vi "ENVIA VALORES-SERVER.vi"() -> ()   [LabVIEW 2019]
uses:
  Strict_Type_Def_Valores_Instrumentos.ctl
  <vilib>/Utility/file.llb/Read Delimited Spreadsheet (string).vi
  Variaveis_Globais_CLP_Paralelo.vi
  Acionamento_Adquiri.vi
panel:
  in  "DP_Lam_max [mmCA]":bool
  in  "Q_Lam[m³/h]":dbl format="%#_4e"
  in  "Rho_Lam/Rho*":dbl
  in  "Mu*/Mu_Lam":dbl format="%#_4e"
  in  "Q*[m³/h]":dbl
  in  "M_Lam[Kg/h]":dbl
  in  "DP_Lam[mmCA]":dbl format="%#_4e"
  in  "SKM-PI-LAM":dbl format="%#_4e"
  in  "SMA-TI-LAM":dbl
  in  "SMA-PI-LAM":dbl
  in  "SKM-PI-BAR":dbl format="%#_4e"
  in  "SKM-TI-WF":dbl
  in  "SKM-TI-KF":dbl
  in  "SKM-TI-AR_COR":dbl
  in  "JK":dbl format="%#_4e"
  in  "JW":dbl format="%#_4e"
  in  "JL":dbl format="%#_4e"
  in  "JG":dbl
  in  "ADQ":bool
  out "size(s)":i32
  in  "SKM-FC-WF_MAX":dbl
  in  "SKM-FC-WF_MIN":dbl
  in  "SKM-PC-TQ_MAX":dbl
  in  "SKM-PC-TQ_MIN":dbl
  in  "SKM-FC-AR_MAX":dbl
  in  "SKM-FC-AR_MIN":dbl
  in  "SKM-FC-KF_MAX":dbl
  in  "SKM-FC-KF_MIN":dbl
  in  "SPK-WR-VEL_MAX":dbl
  in  "SPK-WR-VEL_MIN":dbl
  in  "SPW-WR-VEL_MIN":dbl
  in  "SPW-WR-VEL_MAX":dbl
  in  "SPK-INV-001_ON":bool
  in  "SPK-INV-001_OFF":bool
  in  "SPK-NC-CV-001":bool
  in  "SPK-NC-CV-002":bool
  in  "SPK-NC-CV-003":bool
  in  "SPK-NO-CV-005":bool
  in  "SPK-NC-CV-004":bool
  in  "SPK-NO-CV-006":bool
  in  "SPK-NO-CV-008":bool
  in  "SPK-NO-CV-007":bool
  in  "SPW-INV-001_OFF":bool
  in  "SPW-NC-CV-002":bool
  in  "SPW-INV-001_ON":bool
  in  "SPW-NC-CV-003":bool
  in  "SPW-NO-CV-006":bool
  in  "SPW-NC-CV-001":bool
  in  "SPW-NO-CV-005":bool
  in  "SPW-NO-CV-008":bool
  in  "SPW-NC-CV-004":bool
  in  "SPW-NO-CV-007":bool
  in  "SPW-WR-VEL":dbl
  in  "SPK-WR-VEL":dbl
  in  "SKM-NC-CV_COR":bool
  in  "SKM-NC-CV-JMP":bool
  in  "SKM-NC-CV-LAM":bool
  in  "SKM-FC-AR":dbl
  in  "SKM-FC-KF":dbl
  in  "SKM-FC-WF":dbl
  in  "SKM-PC-TQ":dbl
  in  "PC-TQ-ON":bool
  in  "SKM-AI-KF_COR":dbl
  in  "Diametro_tubulacao":dbl
  in  "SKM-FIC-KF_COR":dbl
  in  "SKM-FI-WF":dbl
  in  "SIA-NC-CV-001":bool
  in  "SIK-NC-CV-001":bool
  in  "SIK-NC-CV-002":bool
  in  "SIT-NC-CV-001":bool
  in  "SIT-NC-CV-002":bool
  in  "SIW-NC-CV-001":bool
  in  "SIW-NC-CV-002":bool
  in  "SKS-NC-CV-001":bool
  in  "SKS-NC-CV-002":bool
  in  "SKS-NC-CV-003":bool
  in  "SKS-NC-CV-004":bool
  in  "SKS-NC-CV-005":bool
  in  "SKS-NC-CV-006":bool
  in  "Valores_Instrumentos":T1 {"JG_AR" format="%#_6e"; "DeltaP_K" format="%#_6e"; "DeltaP_W" format="%#_6e"; "Diâmetro Tubulação [m]" format="%#_6e"; "PC-TQ-TD" format="%#_6e"; "PC-TQ-TI" format="%#_6e"; "PC-TQ-GP" format="%#_6e"; "PC-TQ-PV" format="%#_6e"; "PC-TQ-SP" format="%#_6e"; "PC-TQ-OV" format="%#_6e"; "SPW-WR-VEL" format="%#_6e"; "SPK-WR-VEL" format="%#_6e"; "SKM-PC-TQ" format="%#_6e"; "SKM-FC-KF" format="%#_6e"; "SKM-FC-WF" format="%#_6e"; "SKM-FC-AR" format="%#_6e"; "SKM-TI-KF_COR" format="%#_6e"; "SKS-LC-K" format="%#_6e"; "SPK-RD-CRT" format="%#_6e"; "SPW-RD-CRT" format="%#_6e"; "SKM-FIC-AR_COR" format="%#_6e"; "SKM-FIC-KF_COR" format="%#_6e"; "SKM-AI-AR_COR" format="%#_6e"; "SKM-AI-KF_COR" format="%#_6e"; "SKM-TI-AR_COR" format="%#_6e"; "SKM-TI-KF" format="%#_6e"; "SPW-RD-VEL" format="%#_6e"; "SPK-RD-VEL" format="%#_6e"; "SKS-LC-W" format="%#_6e"; "SIT-PI-002" format="%#_6e"; "SKM-FI-WF" format="%#_6e"; "SKM-TI-WF" format="%#_6e"; "SKM-PI-BAR" format="%#_6e"; "SKM-PI-LAM" format="%#_6e"; "SMA-PI-LAM" format="%#_6e"; "SMA-TI-LAM" format="%#_6e"; "SKM-PI-TQ" format="%#_6e"; "SKM-TI-TQ" format="%#_6e"}
  in  "stop":bool
  in  "VALORES VAZIOS":string[](array[string])
  out "RAN":dbl
  in  "FRA":string
  in  "FLO":dbl
  in  "NUM":i32
  in  "BOTAO":bool
  in  "NOMES":string[](array[string])
  out "Controles":cluster{refnum<vi>[]}
  out "VALORES":string[](array[string])
  # "SKID MEDI敲O - LEITURA"
  # "SKID MEDI敲O - ESCRITA"
  # "SKID BOMBA - ESCRITA"
  # "SKID BOMBA - LEITURA"
  # "SKID SEPARA敲O - LEITURA"
  # "SKID INJE敲O - LEITURA"
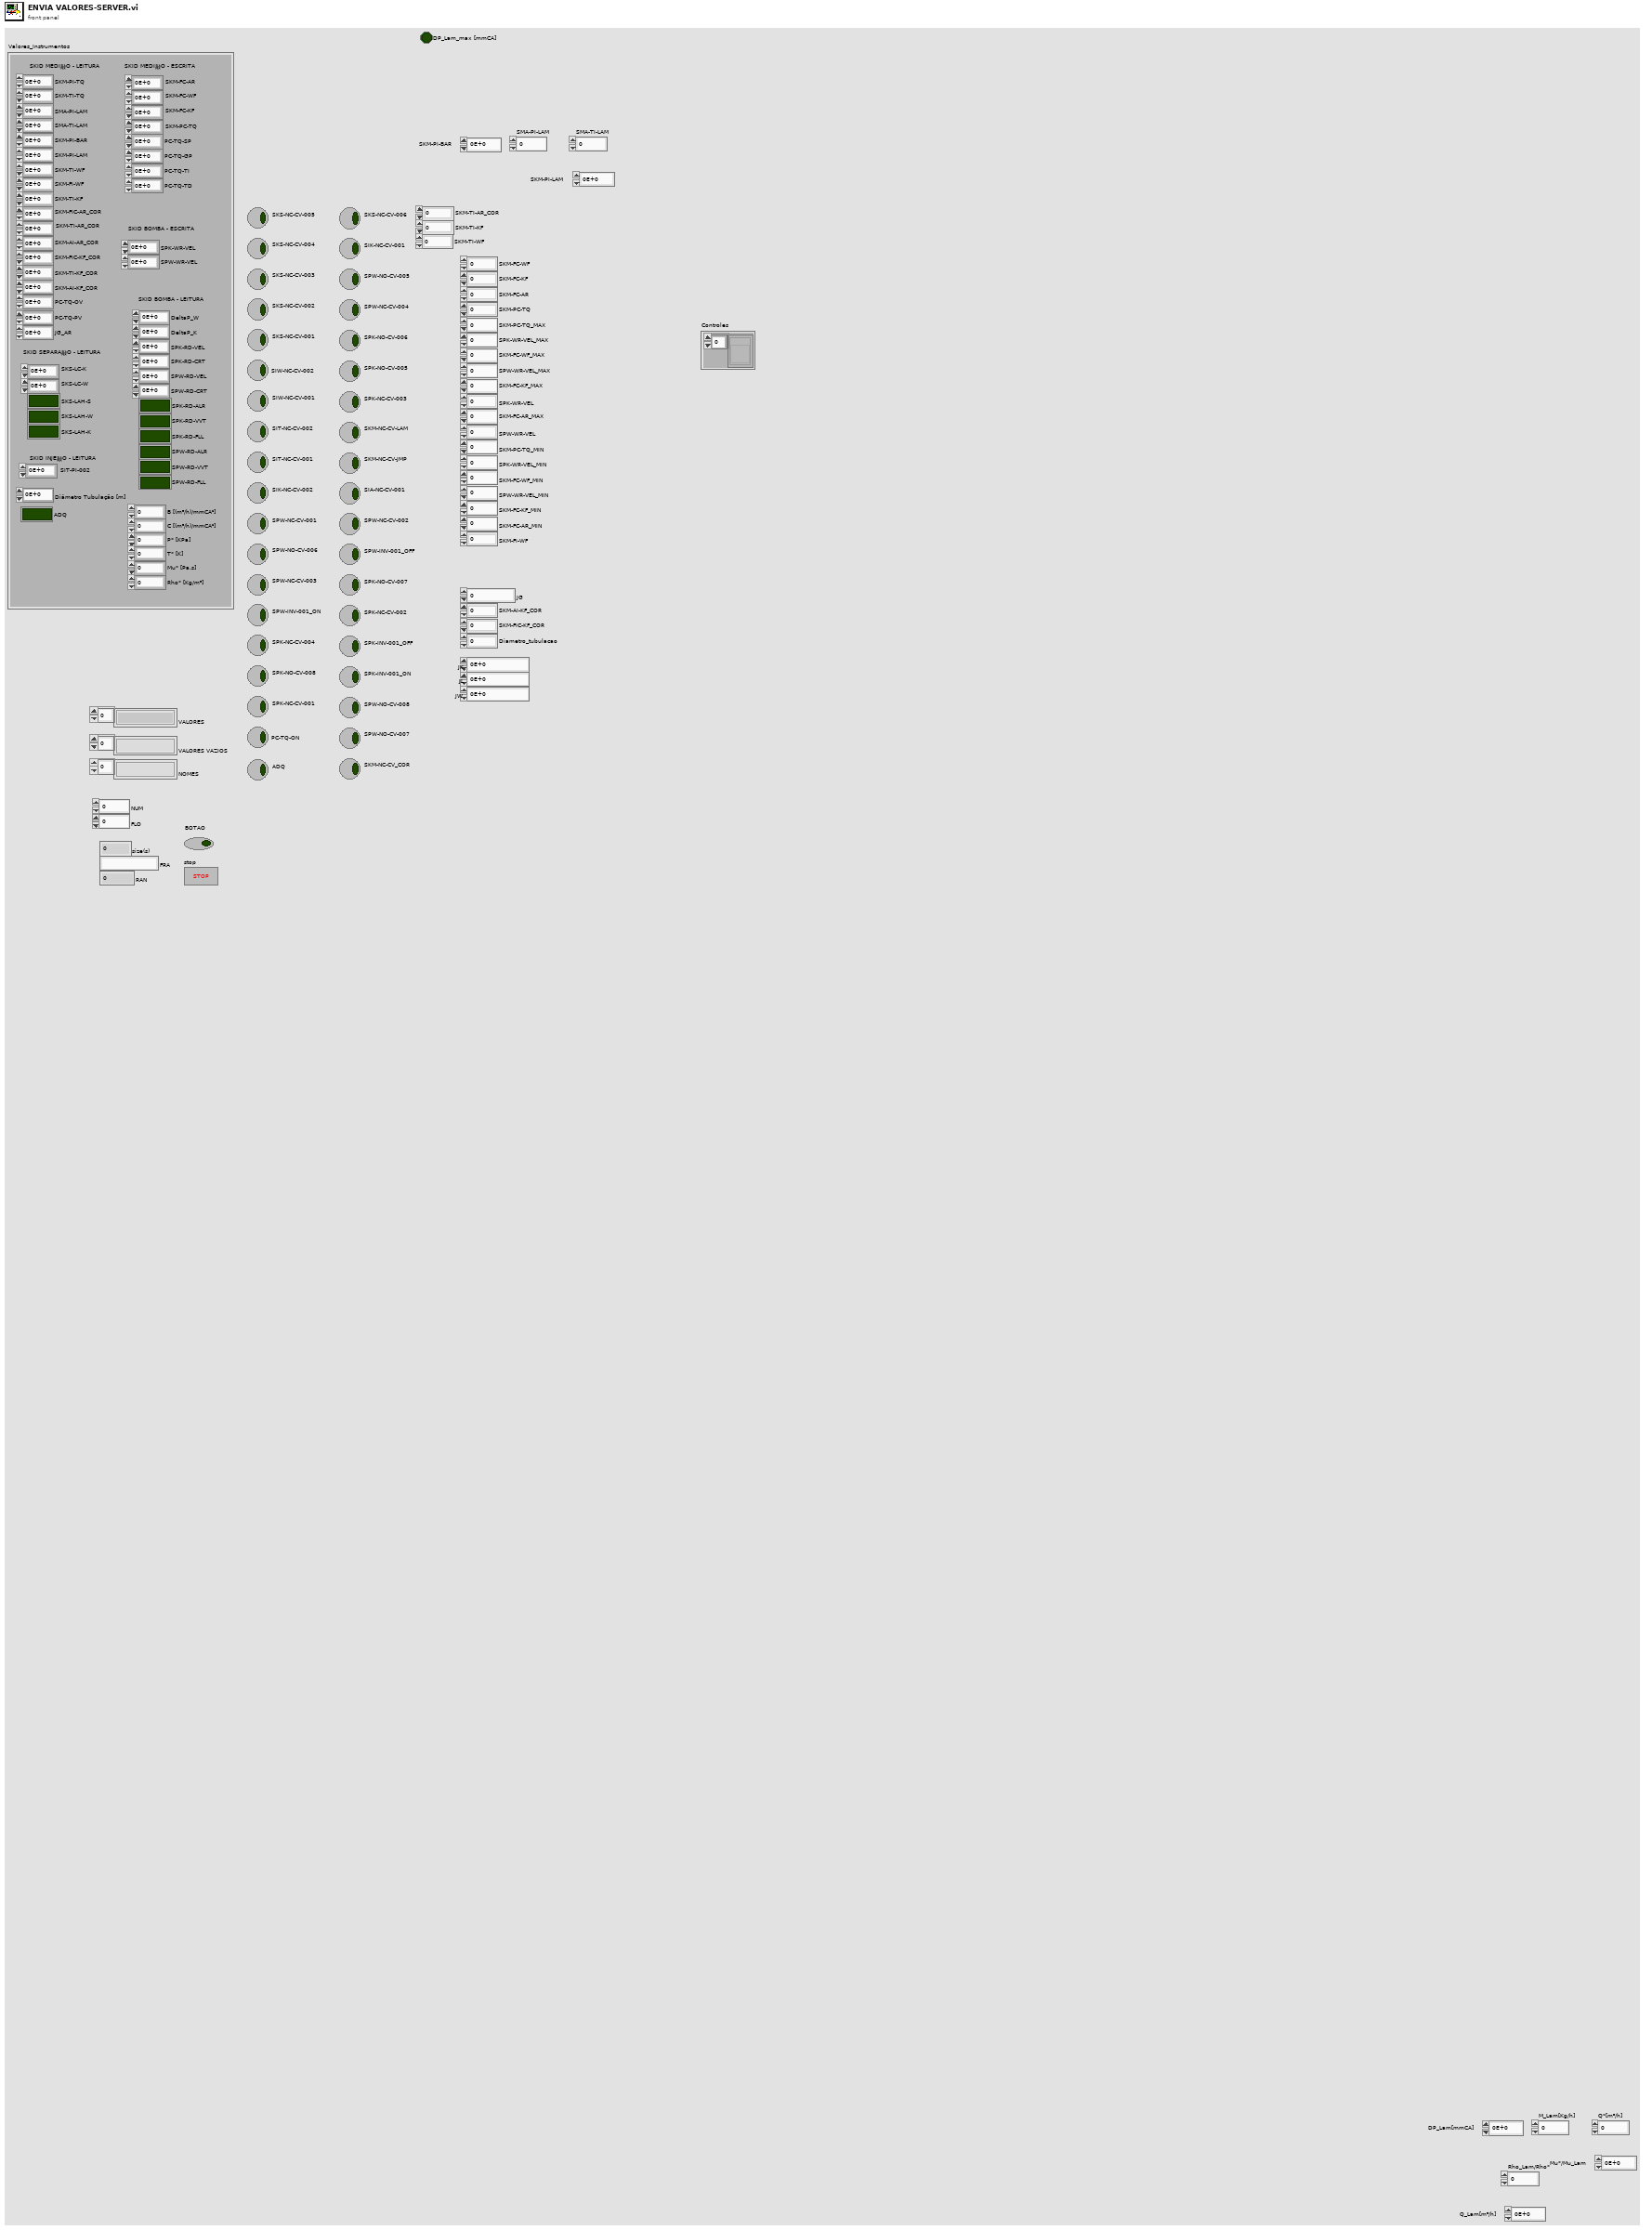
[diagram p1: front panel]
types:
  T1 = typedef "Strict_Type_Def_Valores_Instrumentos.ctl" = cluster{"SKM-TI-TQ":dbl, "SKM-PI-TQ":dbl, "SMA-TI-LAM":dbl, "SMA-PI-LAM":dbl, "SKM-PI-LAM":dbl, "SKM-PI-BAR":dbl, "SKM-TI-WF":dbl, "SKM-FI-WF":dbl, "SIT-PI-002":dbl, "SKS-LC-W":dbl, "SPK-RD-VEL":dbl, "SPW-RD-VEL":dbl, "SKM-TI-KF":dbl, "SKM-TI-AR_COR":dbl, "SKM-AI-KF_COR":dbl, "SKM-AI-AR_COR":dbl, "SKM-FIC-KF_COR":dbl, "SKM-FIC-AR_COR":dbl, "SPW-RD-CRT":dbl, "SPK-RD-CRT":dbl, "SKS-LC-K":dbl, "SKM-TI-KF_COR":dbl, "SKM-FC-AR":dbl, "SKM-FC-WF":dbl, "SKM-FC-KF":dbl, "SKM-PC-TQ":dbl, "SPK-WR-VEL":dbl, "SPW-WR-VEL":dbl, "SPK-RD-ALR":bool, "SPK-RD-VVT":bool, "SPK-RD-FLL":bool, "SPW-RD-ALR":bool, "SPW-RD-VVT":bool, "SPW-RD-FLL":bool, "PC-TQ-OV":dbl, "PC-TQ-SP":dbl, "PC-TQ-PV":dbl, "PC-TQ-GP":dbl, "PC-TQ-TI":dbl, "PC-TQ-TD":dbl, "SKS-LAH-S":bool, "SKS-LAH-W":bool, "SKS-LAH-K":bool, "Diâmetro Tubulação [m]":dbl, "DeltaP_W":dbl, "DeltaP_K":dbl, "ADQ":bool, "JG_AR":dbl, "B [(m³/h)/mmCA²]":dbl, "C [(m³/h)/mmCA²]":dbl, "P* [KPa]":dbl, "T* [K]":dbl, "Mu* [Pa.s] ":dbl, "Rho* [Kg/m³]":dbl}
  T2 = cluster{"Application Name":string, "Description":string, "SPK-NC-CV-001":bool, "SPK-NC-CV-002":bool, "SPK-NC-CV-003":bool, "SPK-NC-CV-004":bool, "SPK-NO-CV-005":bool, "SPK-NO-CV-006":bool, "SPK-NO-CV-007":bool, "SPK-NO-CV-008":bool, "SPK-INV-001":bool, "SPW-NC-CV-001":bool, "SPW-NC-CV-002":bool, "SPW-NC-CV-003":bool, "SPW-NC-CV-004":bool, "SPW-NO-CV-005":bool, "SPW-NO-CV-006":bool, "SPW-NO-CV-007":bool, "SPW-NO-CV-008":bool, "SPW-INV-001":bool, "SKM-NC-CV-LAM":bool, "SKM-NC-CV-COR":bool, "SKM-FV-AR":bool, "SKM-PV-TQ":bool, "SKM-NC-CV-JMP":bool, "SKM-FV-WF":bool, "SKM-FV-KF":bool, "SIW-NC-CV-001":bool, "SIA-NC-CV-001":bool, "SIK-NC-CV-001":bool, "SIT-NC-CV-002":bool, "SIT-NC-CV-001":bool, "SIK-NC-CV-002":bool, "SIW-NC-CV-002":bool, "SKS-NC-CV-001":bool, "SKS-NC-CV-002":bool, "SKS-NC-CV-003":bool, "Boolean":bool, "Boolean 2":bool, "SKS-NC-CV-006":bool}
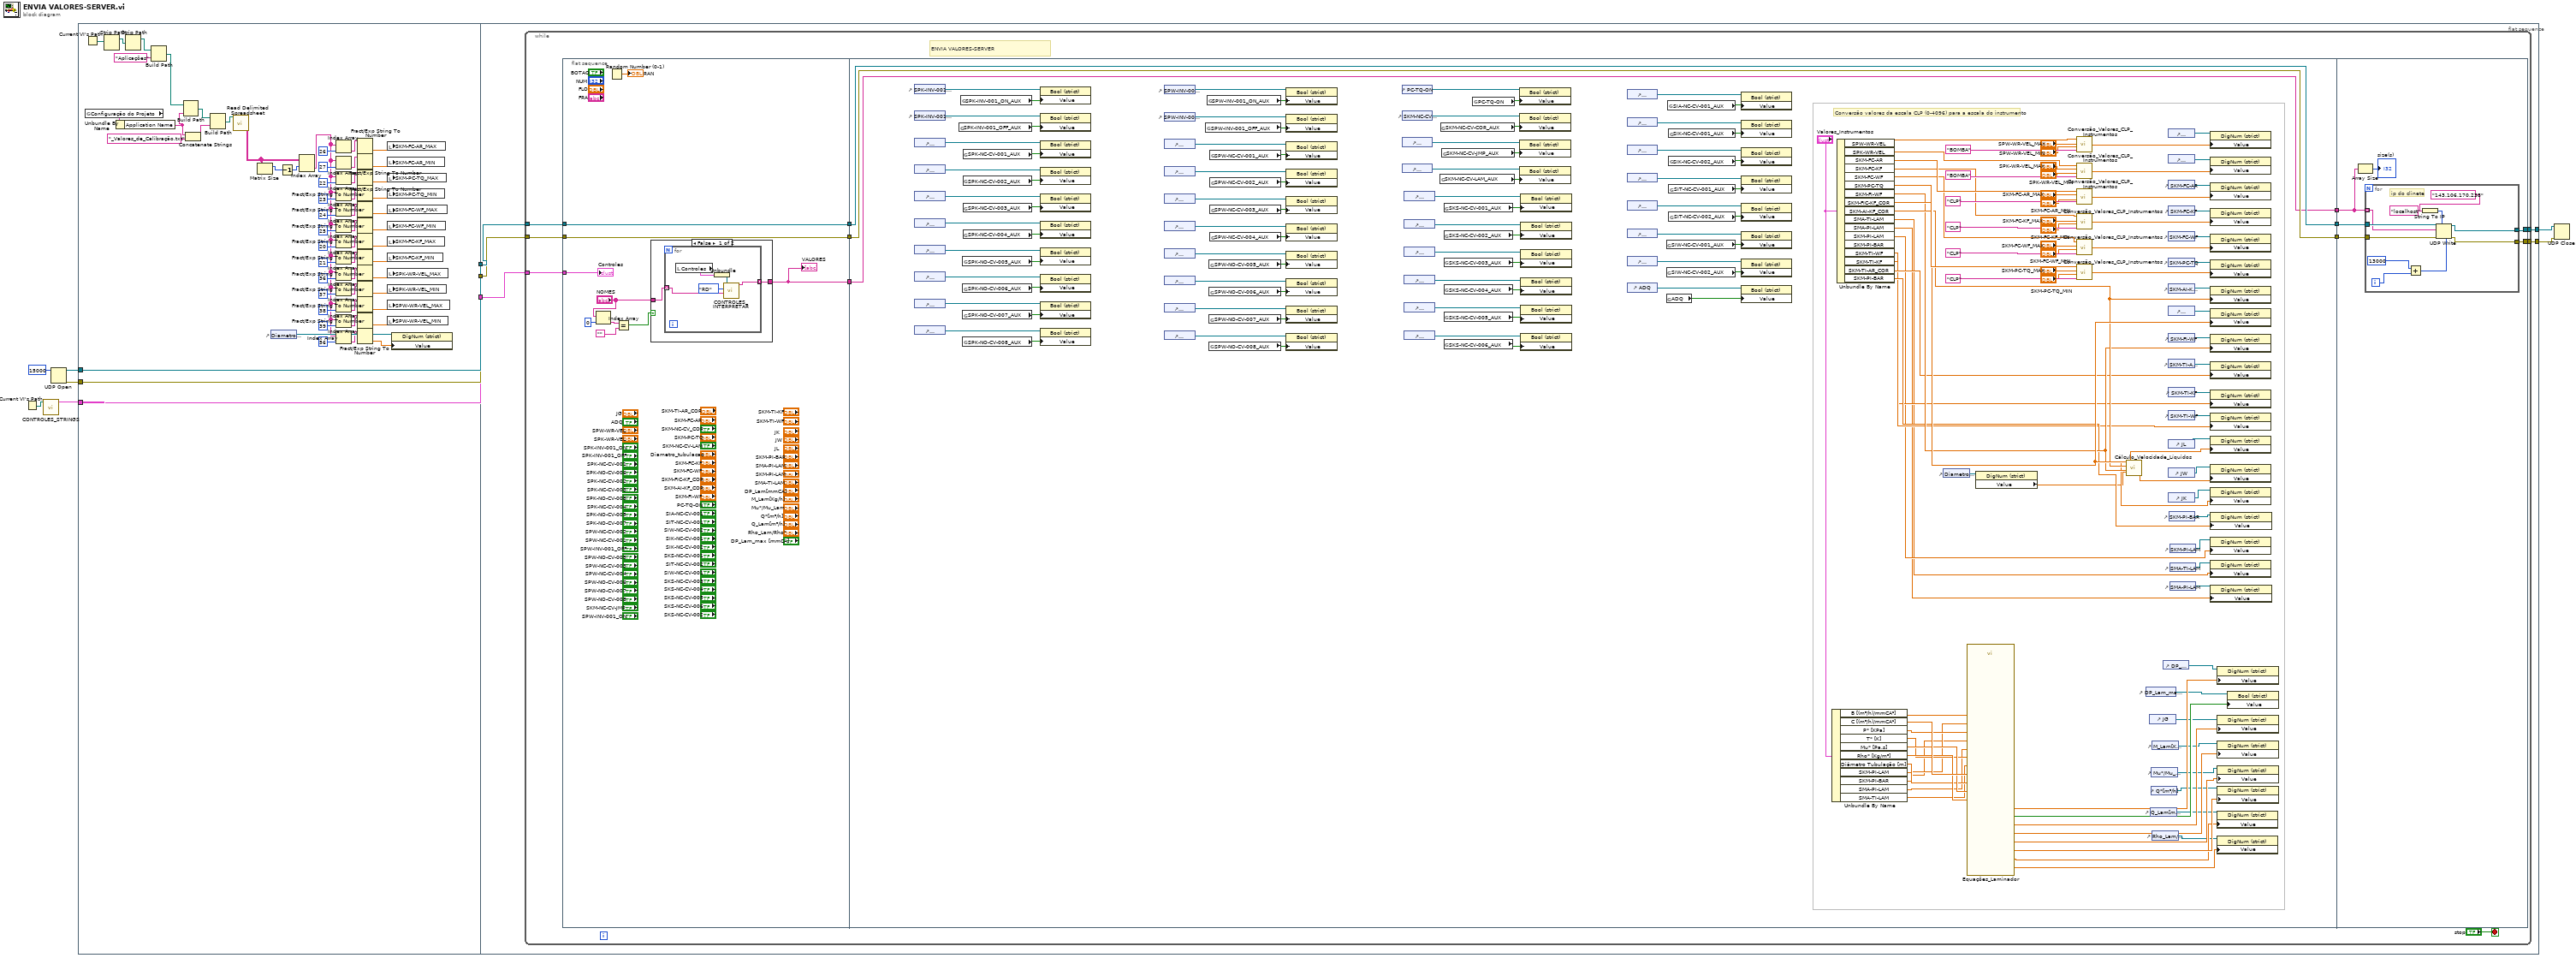
[diagram p0: block diagram]
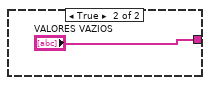
[diagram p2: hidden frame]
diagram:
  n1 = Current VI's Path() -> (path=w7:path)
  n2 = call "CONTROLES_STRINGS.vi"("vi path"=w7) -> ("output cluster"=w6:cluster{refnum<vi>[]})  [unwired: 9 in, 1 out]
  n3 = UDP Open(11:u16 15000 ("port")) -> (port=w9:refnum<k16>, 0:w8:errorcluster)  [unwired: 4 in, 1 out]
  n4 = flat-sequence {
    tunnel: w6 -> [w66]
    tunnel: w8 -> [w67]
    tunnel: w9 -> [w68]
    tunnel: [w68] -> w5
    tunnel: [w67] -> w4
    tunnel: [w66] -> w3
    tunnel: w5 -> [w70]
    tunnel: w4 -> [w69]
    tunnel: w3 -> [w73]
    tunnel: [w72] -> w2
    tunnel: [w71] -> w1
    frame #0 {
      n5 = Current VI's Path() -> (path=w65:path)
      n6 = global read "Variaveis_Globais_para_Configurar_Aplicação_Paralelo.vi" "Configuração do Projeto"() -> (w60:T2)
      n7 = Strip Path(path=w65) -> (stripped path=w64:path)  [unwired: 1 out]
      n8 = Unbundle By Name(w60) -> ("Application Name"=w57:string)
      n9 = Strip Path(path=w64) -> (stripped path=w63:path)  [unwired: 1 out]
      n10 = Build Path(base path=w63, name or relative path="Aplicações") -> (appended path=w61:path)
      n11 = Build Path(base path=w61, name or relative path=w57) -> (appended path=w59:path)
      n12 = Concatenate Strings(w57, "_Valores_de_Calibração.txt" ("string")) -> (w58:string)
      n13 = Build Path(base path=w59, name or relative path=w58) -> (appended path=w55:path)
      n14 = call-poly <vilib>:"Read Delimited Spreadsheet.vi"("file path (dialog if empty)"=w55) -> ("all rows"=w54:string[][])  [unwired: 9 in, 5 out]
      n15 = Matrix Size(0:w54) -> (1:w17:i32)  [unwired: 1 out]
      n16 = control-ref of="Diametro_tubulacao"() -> (w15:refnum<vi>)
      n17 = Decrement(x=w17) -> (x-1=w16:i32)
      n18 = Index Array(array=w54, index (row)=w16) -> (element=w11:string[])  [unwired: 1 in]
      n19 = Index Array(array=w11, index=26) -> (element=w46:string)
      n20 = Index Array(array=w11, index=27) -> (element=w47:string)
      n21 = Index Array(array=w11, index=22) -> (element=w48:string)
      n22 = Index Array(array=w11, index=23) -> (element=w49:string)
      n23 = Index Array(array=w11, index=24) -> (element=w44:string)
      n24 = Index Array(array=w11, index=25) -> (element=w43:string)
      n25 = Index Array(array=w11, index=20) -> (element=w42:string)
      n26 = Index Array(array=w11, index=21) -> (element=w41:string)
      n27 = Index Array(array=w11, index=36) -> (element=w40:string)
      n28 = Index Array(array=w11, index=37) -> (element=w39:string)
      n29 = Index Array(array=w11, index=38) -> (element=w38:string)
      n30 = Index Array(array=w11, index=39) -> (element=w37:string)
      n31 = Index Array(array=w11, index=56) -> (element=w13:string)
      n32 = Fract/Exp String To Number(string=w46) -> (number=w20:dbl)  [unwired: 3 in, 1 out]
      n33 = Fract/Exp String To Number(string=w47) -> (number=w19:dbl)  [unwired: 3 in, 1 out]
      n34 = Fract/Exp String To Number(string=w48) -> (number=w30:dbl)  [unwired: 3 in, 1 out]
      n35 = Fract/Exp String To Number(string=w49) -> (number=w29:dbl)  [unwired: 3 in, 1 out]
      n36 = Fract/Exp String To Number(string=w44) -> (number=w28:dbl)  [unwired: 3 in, 1 out]
      n37 = Fract/Exp String To Number(string=w43) -> (number=w27:dbl)  [unwired: 3 in, 1 out]
      n38 = Fract/Exp String To Number(string=w42) -> (number=w26:dbl)  [unwired: 3 in, 1 out]
      n39 = Fract/Exp String To Number(string=w41) -> (number=w25:dbl)  [unwired: 3 in, 1 out]
      n40 = Fract/Exp String To Number(string=w40) -> (number=w24:dbl)  [unwired: 3 in, 1 out]
      n41 = Fract/Exp String To Number(string=w39) -> (number=w23:dbl)  [unwired: 3 in, 1 out]
      n42 = Fract/Exp String To Number(string=w38) -> (number=w22:dbl)  [unwired: 3 in, 1 out]
      n43 = Fract/Exp String To Number(string=w37) -> (number=w21:dbl)  [unwired: 3 in, 1 out]
      n44 = Fract/Exp String To Number(string=w13) -> (number=w12:dbl)  [unwired: 3 in, 1 out]
      n45 = local write "SKM-FC-AR_MAX"(w20) -> ()
      n46 = local write "SKM-FC-AR_MIN"(w19) -> ()
      n47 = local write "SKM-PC-TQ_MAX"(w30) -> ()
      n48 = local write "SKM-PC-TQ_MIN"(w29) -> ()
      n49 = local write "SKM-FC-WF_MAX"(w28) -> ()
      n50 = local write "SKM-FC-WF_MIN"(w27) -> ()
      n51 = local write "SKM-FC-KF_MAX"(w26) -> ()
      n52 = local write "SKM-FC-KF_MIN"(w25) -> ()
      n53 = local write "SPK-WR-VEL_MAX"(w24) -> ()
      n54 = local write "SPK-WR-VEL_MIN"(w23) -> ()
      n55 = local write "SPW-WR-VEL_MAX"(w22) -> ()
      n56 = local write "SPW-WR-VEL_MIN"(w21) -> ()
      n57 = property class="DigNum (strict)"(reference=w15, "Value"=w12) -> ()  [unwired: 1 in, 2 out]
    }
    frame #1 {
      n58 = while {
        tunnel: w73 -> [w85]
        tunnel: [w77] -> w72
        tunnel: [w76] -> w71
        tunnel: w70 -> [w75]
        tunnel: w69 -> [w74]
        stop <- "stop" stop-if-true
        # "ENVIA VALORES-SERVER"
        n59 = flat-sequence {
          tunnel: [w95] -> w83
          tunnel: [w94] -> w81
          tunnel: [w93] -> w79
          tunnel: w75 -> [w95]
          tunnel: w74 -> [w94]
          tunnel: w85 -> [w91]
          tunnel: w83 -> [w274]
          tunnel: [w274] -> w82
          tunnel: w81 -> [w273]
          tunnel: [w273] -> w80
          tunnel: w79 -> [w272]
          tunnel: [w272] -> w78
          tunnel: [w278] -> w77
          tunnel: [w277] -> w76
          tunnel: w82 -> [w280]
          tunnel: w80 -> [w279]
          tunnel: w78 -> [w276]
          frame #0 {
            n60 = Index Array(array="NOMES", index=0) -> (element=w88:string)
            n61 = Random Number (0-1)() -> (number: 0 to 1=→"RAN":dbl)
            n62 = Equal?(x=w88, y="") -> (x = y?=w86:bool)
            n63 = case shown="False" w86 {
              tunnel: [w97 "VALORES VAZIOS"] -> w93
              tunnel: "NOMES" -> [w96 _]
              frame False {
                n64 = for {
                  tunnel: w96 -> [w100] mode=indexing
                  tunnel: [w98] -> w97 mode=indexing
                  n65 = local read "Controles"() -> (w102:cluster{refnum<vi>[]})
                  n66 = Unbundle(w102) -> (w101:refnum<vi>[])
                  n67 = call "CONTROLES_INTERPRETAR.vi"("name"=w100, "RD/WR"=enum16{"WR", "RD"}."RD", "Controls[]"=w101) -> ("Data"=w98:string)  [unwired: 6 in, 2 out]
                }
              }
              frame True {
              }
            }
            "VALORES" <- w93
            "Controles" <- w91
          }
          frame #1 {
            # "Conversão valores da escala CLP (0-4096) para a escala do instrumento"
            n68 = control-ref of="SPK-INV-001_ON"() -> (w253:refnum<vi>)
            n69 = control-ref of="SPK-INV-001_OFF"() -> (w254:refnum<vi>)
            n70 = control-ref of="SPK-NC-CV-001"() -> (w255:refnum<vi>)
            n71 = control-ref of="SPK-NC-CV-002"() -> (w256:refnum<vi>)
            n72 = control-ref of="SPK-NC-CV-003"() -> (w257:refnum<vi>)
            n73 = control-ref of="SPK-NC-CV-004"() -> (w259:refnum<vi>)
            n74 = control-ref of="SPK-NO-CV-005"() -> (w258:refnum<vi>)
            n75 = control-ref of="SPK-NO-CV-006"() -> (w260:refnum<vi>)
            n76 = control-ref of="SPK-NO-CV-007"() -> (w262:refnum<vi>)
            n77 = control-ref of="SPK-NO-CV-008"() -> (w261:refnum<vi>)
            n78 = global read "Variaveis_Globais_CLP_Paralelo.vi" "SPK-INV-001_OFF_AUX"() -> (w270:bool)
            n79 = global read "Variaveis_Globais_CLP_Paralelo.vi" "SPK-INV-001_ON_AUX"() -> (w271:bool)
            n80 = global read "Variaveis_Globais_CLP_Paralelo.vi" "SPK-NO-CV-005_AUX"() -> (w265:bool)
            n81 = global read "Variaveis_Globais_CLP_Paralelo.vi" "SPK-NO-CV-006_AUX"() -> (w264:bool)
            n82 = global read "Variaveis_Globais_CLP_Paralelo.vi" "SPK-NO-CV-007_AUX"() -> (w263:bool)
            n83 = global read "Variaveis_Globais_CLP_Paralelo.vi" "SPK-NO-CV-008_AUX"() -> (w160:bool)
            n84 = global read "Variaveis_Globais_CLP_Paralelo.vi" "SPK-NC-CV-001_AUX"() -> (w269:bool)
            n85 = global read "Variaveis_Globais_CLP_Paralelo.vi" "SPK-NC-CV-002_AUX"() -> (w268:bool)
            n86 = global read "Variaveis_Globais_CLP_Paralelo.vi" "SPK-NC-CV-003_AUX"() -> (w267:bool)
            n87 = global read "Variaveis_Globais_CLP_Paralelo.vi" "SPK-NC-CV-004_AUX"() -> (w266:bool)
            n88 = property class="Bool (strict)"(reference=w253, "Value"=w271) -> ()  [unwired: 1 in, 2 out]
            n89 = property class="Bool (strict)"(reference=w254, "Value"=w270) -> ()  [unwired: 1 in, 2 out]
            n90 = property class="Bool (strict)"(reference=w255, "Value"=w269) -> ()  [unwired: 1 in, 2 out]
            n91 = property class="Bool (strict)"(reference=w256, "Value"=w268) -> ()  [unwired: 1 in, 2 out]
            n92 = property class="Bool (strict)"(reference=w257, "Value"=w267) -> ()  [unwired: 1 in, 2 out]
            n93 = property class="Bool (strict)"(reference=w259, "Value"=w266) -> ()  [unwired: 1 in, 2 out]
            n94 = property class="Bool (strict)"(reference=w258, "Value"=w265) -> ()  [unwired: 1 in, 2 out]
            n95 = property class="Bool (strict)"(reference=w260, "Value"=w264) -> ()  [unwired: 1 in, 2 out]
            n96 = property class="Bool (strict)"(reference=w262, "Value"=w263) -> ()  [unwired: 1 in, 2 out]
            n97 = property class="Bool (strict)"(reference=w261, "Value"=w160) -> ()  [unwired: 1 in, 2 out]
            n98 = control-ref of="SPW-INV-001_ON"() -> (w235:refnum<vi>)
            n99 = control-ref of="SPW-INV-001_OFF"() -> (w233:refnum<vi>)
            n100 = control-ref of="SPW-NC-CV-001"() -> (w238:refnum<vi>)
            n101 = control-ref of="SPW-NC-CV-002"() -> (w234:refnum<vi>)
            n102 = control-ref of="SPW-NC-CV-003"() -> (w236:refnum<vi>)
            n103 = control-ref of="SPW-NC-CV-004"() -> (w241:refnum<vi>)
            n104 = control-ref of="SPW-NO-CV-005"() -> (w239:refnum<vi>)
            n105 = control-ref of="SPW-NO-CV-006"() -> (w237:refnum<vi>)
            n106 = control-ref of="SPW-NO-CV-007"() -> (w242:refnum<vi>)
            n107 = control-ref of="SPW-NO-CV-008"() -> (w240:refnum<vi>)
            n108 = global read "Variaveis_Globais_CLP_Paralelo.vi" "SPW-INV-001_OFF_AUX"() -> (w243:bool)
            n109 = global read "Variaveis_Globais_CLP_Paralelo.vi" "SPW-INV-001_ON_AUX"() -> (w245:bool)
            n110 = global read "Variaveis_Globais_CLP_Paralelo.vi" "SPW-NO-CV-005_AUX"() -> (w249:bool)
            n111 = global read "Variaveis_Globais_CLP_Paralelo.vi" "SPW-NO-CV-006_AUX"() -> (w247:bool)
            n112 = global read "Variaveis_Globais_CLP_Paralelo.vi" "SPW-NO-CV-007_AUX"() -> (w252:bool)
            n113 = global read "Variaveis_Globais_CLP_Paralelo.vi" "SPW-NO-CV-008_AUX"() -> (w250:bool)
            n114 = global read "Variaveis_Globais_CLP_Paralelo.vi" "SPW-NC-CV-001_AUX"() -> (w248:bool)
            n115 = global read "Variaveis_Globais_CLP_Paralelo.vi" "SPW-NC-CV-002_AUX"() -> (w244:bool)
            n116 = global read "Variaveis_Globais_CLP_Paralelo.vi" "SPW-NC-CV-003_AUX"() -> (w246:bool)
            n117 = global read "Variaveis_Globais_CLP_Paralelo.vi" "SPW-NC-CV-004_AUX"() -> (w251:bool)
            n118 = property class="Bool (strict)"(reference=w235, "Value"=w245) -> ()  [unwired: 1 in, 2 out]
            n119 = property class="Bool (strict)"(reference=w233, "Value"=w243) -> ()  [unwired: 1 in, 2 out]
            n120 = property class="Bool (strict)"(reference=w238, "Value"=w248) -> ()  [unwired: 1 in, 2 out]
            n121 = property class="Bool (strict)"(reference=w234, "Value"=w244) -> ()  [unwired: 1 in, 2 out]
            n122 = property class="Bool (strict)"(reference=w236, "Value"=w246) -> ()  [unwired: 1 in, 2 out]
            n123 = property class="Bool (strict)"(reference=w241, "Value"=w251) -> ()  [unwired: 1 in, 2 out]
            n124 = property class="Bool (strict)"(reference=w239, "Value"=w249) -> ()  [unwired: 1 in, 2 out]
            n125 = property class="Bool (strict)"(reference=w237, "Value"=w247) -> ()  [unwired: 1 in, 2 out]
            n126 = property class="Bool (strict)"(reference=w242, "Value"=w252) -> ()  [unwired: 1 in, 2 out]
            n127 = property class="Bool (strict)"(reference=w240, "Value"=w250) -> ()  [unwired: 1 in, 2 out]
            n128 = control-ref of="PC-TQ-ON"() -> (w228:refnum<vi>)
            n129 = control-ref of="SKM-NC-CV_COR"() -> (w225:refnum<vi>)
            n130 = control-ref of="SKM-NC-CV-JMP"() -> (w226:refnum<vi>)
            n131 = control-ref of="SKM-NC-CV-LAM"() -> (w227:refnum<vi>)
            n132 = control-ref of="SKS-NC-CV-001"() -> (w214:refnum<vi>)
            n133 = control-ref of="SKS-NC-CV-002"() -> (w215:refnum<vi>)
            n134 = control-ref of="SKS-NC-CV-003"() -> (w216:refnum<vi>)
            n135 = control-ref of="SKS-NC-CV-004"() -> (w217:refnum<vi>)
            n136 = control-ref of="SKS-NC-CV-005"() -> (w218:refnum<vi>)
            n137 = control-ref of="SKS-NC-CV-006"() -> (w213:refnum<vi>)
            n138 = global read "Variaveis_Globais_CLP_Paralelo.vi" "SKM-NC-CV-LAM_AUX"() -> (w229:bool)
            n139 = global read "Variaveis_Globais_CLP_Paralelo.vi" "SKM-NC-CV-COR_AUX"() -> (w231:bool)
            n140 = global read "Variaveis_Globais_CLP_Paralelo.vi" "SKM-NC-CV-JMP_AUX"() -> (w230:bool)
            n141 = global read "Variaveis_Globais_CLP_Paralelo.vi" "SKS-NC-CV-001_AUX"() -> (w219:bool)
            n142 = global read "Variaveis_Globais_CLP_Paralelo.vi" "SKS-NC-CV-002_AUX"() -> (w224:bool)
            n143 = global read "Variaveis_Globais_CLP_Paralelo.vi" "SKS-NC-CV-003_AUX"() -> (w223:bool)
            n144 = global read "Variaveis_Globais_CLP_Paralelo.vi" "SKS-NC-CV-004_AUX"() -> (w222:bool)
            n145 = global read "Variaveis_Globais_CLP_Paralelo.vi" "SKS-NC-CV-005_AUX"() -> (w221:bool)
            n146 = global read "Variaveis_Globais_CLP_Paralelo.vi" "SKS-NC-CV-006_AUX"() -> (w220:bool)
            n147 = global read "Variaveis_Globais_CLP_Paralelo.vi" "PC-TQ-ON"() -> (w232:bool)
            n148 = property class="Bool (strict)"(reference=w228, "Value"=w232) -> ()  [unwired: 1 in, 2 out]
            n149 = property class="Bool (strict)"(reference=w225, "Value"=w231) -> ()  [unwired: 1 in, 2 out]
            n150 = property class="Bool (strict)"(reference=w226, "Value"=w230) -> ()  [unwired: 1 in, 2 out]
            n151 = property class="Bool (strict)"(reference=w227, "Value"=w229) -> ()  [unwired: 1 in, 2 out]
            n152 = property class="Bool (strict)"(reference=w214, "Value"=w219) -> ()  [unwired: 1 in, 2 out]
            n153 = property class="Bool (strict)"(reference=w215, "Value"=w224) -> ()  [unwired: 1 in, 2 out]
            n154 = property class="Bool (strict)"(reference=w216, "Value"=w223) -> ()  [unwired: 1 in, 2 out]
            n155 = property class="Bool (strict)"(reference=w217, "Value"=w222) -> ()  [unwired: 1 in, 2 out]
            n156 = property class="Bool (strict)"(reference=w218, "Value"=w221) -> ()  [unwired: 1 in, 2 out]
            n157 = property class="Bool (strict)"(reference=w213, "Value"=w220) -> ()  [unwired: 1 in, 2 out]
            n158 = control-ref of="SIA-NC-CV-001"() -> (w199:refnum<vi>)
            n159 = control-ref of="SIK-NC-CV-001"() -> (w200:refnum<vi>)
            n160 = control-ref of="SIK-NC-CV-002"() -> (w201:refnum<vi>)
            n161 = control-ref of="SIT-NC-CV-001"() -> (w202:refnum<vi>)
            n162 = control-ref of="SIT-NC-CV-002"() -> (w203:refnum<vi>)
            n163 = control-ref of="SIW-NC-CV-001"() -> (w204:refnum<vi>)
            n164 = control-ref of="SIW-NC-CV-002"() -> (w205:refnum<vi>)
            n165 = control-ref of="ADQ"() -> (w159:refnum<vi>)
            n166 = global read "Variaveis_Globais_CLP_Paralelo.vi" "SIW-NC-CV-001_AUX"() -> (w207:bool)
            n167 = global read "Variaveis_Globais_CLP_Paralelo.vi" "SIW-NC-CV-002_AUX"() -> (w206:bool)
            n168 = global read "Acionamento_Adquiri.vi" "ADQ"() -> (w158:bool)
            n169 = global read "Variaveis_Globais_CLP_Paralelo.vi" "SIA-NC-CV-001_AUX"() -> (w212:bool)
            n170 = global read "Variaveis_Globais_CLP_Paralelo.vi" "SIK-NC-CV-001_AUX"() -> (w211:bool)
            n171 = global read "Variaveis_Globais_CLP_Paralelo.vi" "SIK-NC-CV-002_AUX"() -> (w210:bool)
            n172 = global read "Variaveis_Globais_CLP_Paralelo.vi" "SIT-NC-CV-001_AUX"() -> (w209:bool)
            n173 = global read "Variaveis_Globais_CLP_Paralelo.vi" "SIT-NC-CV-002_AUX"() -> (w208:bool)
            n174 = property class="Bool (strict)"(reference=w199, "Value"=w212) -> ()  [unwired: 1 in, 2 out]
            n175 = property class="Bool (strict)"(reference=w200, "Value"=w211) -> ()  [unwired: 1 in, 2 out]
            n176 = property class="Bool (strict)"(reference=w201, "Value"=w210) -> ()  [unwired: 1 in, 2 out]
            n177 = property class="Bool (strict)"(reference=w202, "Value"=w209) -> ()  [unwired: 1 in, 2 out]
            n178 = property class="Bool (strict)"(reference=w203, "Value"=w208) -> ()  [unwired: 1 in, 2 out]
            n179 = property class="Bool (strict)"(reference=w204, "Value"=w207) -> ()  [unwired: 1 in, 2 out]
            n180 = property class="Bool (strict)"(reference=w205, "Value"=w206) -> ()  [unwired: 1 in, 2 out]
            n181 = property class="Bool (strict)"(reference=w159, "Value"=w158) -> ()  [unwired: 1 in, 2 out]
            n182 = Unbundle By Name("Valores_Instrumentos") -> ("B [(m³/h)/mmCA²]"=w131:dbl, "C [(m³/h)/mmCA²]"=w130:dbl, "P* [KPa]"=w124:dbl, "T* [K]"=w125:dbl, "Mu* [Pa.s]"=w128:dbl, "Rho* [Kg/m³]"=w129:dbl, "Diâmetro Tubulação [m]"=w127:dbl, "SKM-PI-LAM"=w123:dbl, "SKM-PI-BAR"=w122:dbl, "SMA-PI-LAM"=w121:dbl, "SMA-TI-LAM"=w120:dbl)
            n183 = Unbundle By Name("Valores_Instrumentos") -> ("SPW-WR-VEL"=w188:dbl, "SPK-WR-VEL"=w165:dbl, "SKM-FC-AR"=w164:dbl, "SKM-FC-KF"=w163:dbl, "SKM-FC-WF"=w162:dbl, "SKM-PC-TQ"=w161:dbl, "SKM-FI-WF"=w155:dbl, "SKM-FIC-KF_COR"=w157:dbl, "SKM-AI-KF_COR"=w156:dbl, "SMA-TI-LAM"=w134:dbl, "SMA-PI-LAM"=w133:dbl, "SKM-PI-LAM"=w135:dbl, "SKM-TI-WF"=w140:dbl, "SKM-TI-KF"=w139:dbl, "SKM-TI-AR_COR"=w149:dbl, "SKM-PI-BAR"=w141:dbl)  [unwired: 1 out]
            n184 = control-ref of="Diametro_tubulacao"() -> (w154:refnum<vi>)
            n185 = call "Equações_Laminador.vi"("DP_Lam [KPa]"=w123, "B [(m³/h)/mmCA²]"=w131, "C [(m³/h)/mmCA]"=w130, "P* [KPa]"=w124, "T* [K]"=w125, "P_Bar [KPa]"=w122, "P_Lam [KPa]"=w121, "T_Lam [ºC]"=w120, "Rho* [Kg/m³]"=w129, "Mu* [Pa.s]"=w128, "Diâmetro da tubulação [m]"=w127) -> ("DP_Lam [mmCA]"=w119:dbl, "DP_Lam_max [mmCA]"=w116:bool, "M_Lam [Kg/h]"=w112:dbl, "Q* [m³/h]"=w108:dbl, "Q_Lam [m³/h]"=w106:dbl, "Jg [m/s]"=w114:dbl, "Mu*/Mu_Lam"=w110:dbl, "Rho_Nist/Rho*"=w104:dbl)  [unwired: 9 in]
            n186 = property class="DigNum (strict)"(reference=w154) -> ("Value"=w126:dbl)  [unwired: 1 in, 2 out]
            n187 = call "Conversão_Valores_CLP_Instrumentos.vi"("String"="BOMBA", "MIN"="SPW-WR-VEL_MIN", "MAX"="SPW-WR-VEL_MAX", "CLP"=w188) -> ("S"=w182:dbl)
            n188 = call "Conversão_Valores_CLP_Instrumentos.vi"("String"="BOMBA", "MIN"="SPK-WR-VEL_MIN", "MAX"="SPK-WR-VEL_MAX", "CLP"=w165) -> ("S"=w181:dbl)
            n189 = call "Conversão_Valores_CLP_Instrumentos.vi"("String"="CLP", "MIN"="SKM-FC-AR_MIN", "MAX"="SKM-FC-AR_MAX", "CLP"=w164) -> ("S"=w180:dbl)
            n190 = call "Conversão_Valores_CLP_Instrumentos.vi"("String"="CLP", "MIN"="SKM-FC-KF_MIN", "MAX"="SKM-FC-KF_MAX", "CLP"=w163) -> ("S"=w179:dbl)
            n191 = call "Conversão_Valores_CLP_Instrumentos.vi"("String"="CLP", "MIN"="SKM-FC-WF_MIN", "MAX"="SKM-FC-WF_MAX", "CLP"=w162) -> ("S"=w178:dbl)
            n192 = call "Conversão_Valores_CLP_Instrumentos.vi"("String"="CLP", "MIN"="SKM-PC-TQ_MIN", "MAX"="SKM-PC-TQ_MAX", "CLP"=w161) -> ("S"=w152:dbl)
            n193 = call "Cálculo_Velocidade_Líquidos.vi"("Diâmetro Tubulação [m]"=w126, "SKM-FI-WF"=w155, "SKM-AI-KF_COR"=w156, "SKM-FIC-KF_COR"=w157) -> ("Velocidade Líquido [m/s]"=w143:dbl, "Velocidade Água [m/s]"=w145:dbl, "Velocidade Querosene [m/s]"=w147:dbl)  [unwired: 5 in]
            n194 = control-ref of="DP_Lam_max [mmCA]"() -> (w117:refnum<vi>)
            n195 = control-ref of="JG"() -> (w115:refnum<vi>)
            n196 = control-ref of="Q_Lam[m³/h]"() -> (w107:refnum<vi>)
            n197 = control-ref of="Q*[m³/h]"() -> (w109:refnum<vi>)
            n198 = control-ref of="Mu*/Mu_Lam"() -> (w111:refnum<vi>)
            n199 = control-ref of="Rho_Lam/Rho*"() -> (w105:refnum<vi>)
            n200 = control-ref of="M_Lam[Kg/h]"() -> (w113:refnum<vi>)
            n201 = control-ref of="DP_Lam[mmCA]"() -> (w118:refnum<vi>)
            n202 = control-ref of="SPW-WR-VEL"() -> (w190:refnum<vi>)
            n203 = control-ref of="SPK-WR-VEL"() -> (w198:refnum<vi>)
            n204 = control-ref of="SKM-FC-AR"() -> (w191:refnum<vi>)
            n205 = control-ref of="SKM-FC-KF"() -> (w192:refnum<vi>)
            n206 = control-ref of="SKM-FC-WF"() -> (w193:refnum<vi>)
            n207 = control-ref of="SKM-PC-TQ"() -> (w194:refnum<vi>)
            n208 = control-ref of="SKM-AI-KF_COR"() -> (w195:refnum<vi>)
            n209 = control-ref of="SKM-FIC-KF_COR"() -> (w196:refnum<vi>)
            n210 = control-ref of="SKM-FI-WF"() -> (w197:refnum<vi>)
            n211 = control-ref of="SKM-TI-AR_COR"() -> (w153:refnum<vi>)
            n212 = control-ref of="SKM-TI-KF"() -> (w151:refnum<vi>)
            n213 = control-ref of="SKM-TI-WF"() -> (w150:refnum<vi>)
            n214 = control-ref of="JL"() -> (w144:refnum<vi>)
            n215 = control-ref of="JW"() -> (w146:refnum<vi>)
            n216 = control-ref of="JK"() -> (w148:refnum<vi>)
            n217 = control-ref of="SKM-PI-BAR"() -> (w142:refnum<vi>)
            n218 = control-ref of="SKM-PI-LAM"() -> (w138:refnum<vi>)
            n219 = control-ref of="SMA-TI-LAM"() -> (w137:refnum<vi>)
            n220 = control-ref of="SMA-PI-LAM"() -> (w136:refnum<vi>)
            n221 = property class="DigNum (strict)"(reference=w190, "Value"=w182) -> ()  [unwired: 1 in, 2 out]
            n222 = property class="DigNum (strict)"(reference=w198, "Value"=w181) -> ()  [unwired: 1 in, 2 out]
            n223 = property class="DigNum (strict)"(reference=w191, "Value"=w180) -> ()  [unwired: 1 in, 2 out]
            n224 = property class="DigNum (strict)"(reference=w192, "Value"=w179) -> ()  [unwired: 1 in, 2 out]
            n225 = property class="DigNum (strict)"(reference=w193, "Value"=w178) -> ()  [unwired: 1 in, 2 out]
            n226 = property class="DigNum (strict)"(reference=w194, "Value"=w152) -> ()  [unwired: 1 in, 2 out]
            n227 = property class="DigNum (strict)"(reference=w195, "Value"=w156) -> ()  [unwired: 1 in, 2 out]
            n228 = property class="DigNum (strict)"(reference=w196, "Value"=w157) -> ()  [unwired: 1 in, 2 out]
            n229 = property class="DigNum (strict)"(reference=w197, "Value"=w155) -> ()  [unwired: 1 in, 2 out]
            n230 = property class="DigNum (strict)"(reference=w153, "Value"=w149) -> ()  [unwired: 1 in, 2 out]
            n231 = property class="DigNum (strict)"(reference=w151, "Value"=w139) -> ()  [unwired: 1 in, 2 out]
            n232 = property class="DigNum (strict)"(reference=w150, "Value"=w140) -> ()  [unwired: 1 in, 2 out]
            n233 = property class="DigNum (strict)"(reference=w144, "Value"=w143) -> ()  [unwired: 1 in, 2 out]
            n234 = property class="DigNum (strict)"(reference=w146, "Value"=w145) -> ()  [unwired: 1 in, 2 out]
            n235 = property class="DigNum (strict)"(reference=w148, "Value"=w147) -> ()  [unwired: 1 in, 2 out]
            n236 = property class="DigNum (strict)"(reference=w138, "Value"=w135) -> ()  [unwired: 1 in, 2 out]
            n237 = property class="DigNum (strict)"(reference=w137, "Value"=w134) -> ()  [unwired: 1 in, 2 out]
            n238 = property class="DigNum (strict)"(reference=w142, "Value"=w141) -> ()  [unwired: 1 in, 2 out]
            n239 = property class="DigNum (strict)"(reference=w136, "Value"=w133) -> ()  [unwired: 1 in, 2 out]
            n240 = property class="DigNum (strict)"(reference=w107, "Value"=w106) -> ()  [unwired: 1 in, 2 out]
            n241 = property class="DigNum (strict)"(reference=w105, "Value"=w104) -> ()  [unwired: 1 in, 2 out]
            n242 = property class="DigNum (strict)"(reference=w118, "Value"=w119) -> ()  [unwired: 1 in, 2 out]
            n243 = property class="DigNum (strict)"(reference=w115, "Value"=w114) -> ()  [unwired: 1 in, 2 out]
            n244 = property class="DigNum (strict)"(reference=w113, "Value"=w112) -> ()  [unwired: 1 in, 2 out]
            n245 = property class="DigNum (strict)"(reference=w111, "Value"=w110) -> ()  [unwired: 1 in, 2 out]
            n246 = property class="DigNum (strict)"(reference=w109, "Value"=w108) -> ()  [unwired: 1 in, 2 out]
            n247 = property class="Bool (strict)"(reference=w117, "Value"=w116) -> ()  [unwired: 1 in, 2 out]
          }
          frame #2 {
            n248 = Array Size(array=w276) -> (size(s)=→"size(s)":i32)
            n249 = for {
              tunnel: w280 -> [w290]
              tunnel: w279 -> [w289]
              tunnel: w276 -> [w284] mode=indexing
              tunnel: [w283] -> w278
              tunnel: [w282] -> w277
              i -> [w287]
              (unwired) "localhost" ("name")
              # "ip do clinete"
              n250 = Add(x=u16 13000 ("port or service name"), y=w287) -> (x+y=w285:i32)
              n251 = String To IP(1:"143.106.170.238" ("name")) -> (0:w288:u32)
              n252 = UDP Write(address=w288, port or service name=w285, connection ID=w290, data in=w284, 8:w289) -> (error out=w282:errorcluster, 3:w283:refnum<k16>)  [unwired: 1 in]
            }
          }
        }
      }
    }
  }
  n253 = UDP Close(connection ID=w2, 8:w1) -> ()  [unwired: 2 out]
